vi "comm set rts.vi"(8 "error in (no error)":errorcluster, 11 "Comm Handle":u32) -> (0 "error out":errorcluster, 3 "dup Comm Handle":u32)   [LabVIEW 2017, in "lvserial.lvlib"]
doc: "Sends the RTS (RequestToSend) signal."
uses:
  lvserial.lvlib
  lvserial.dll
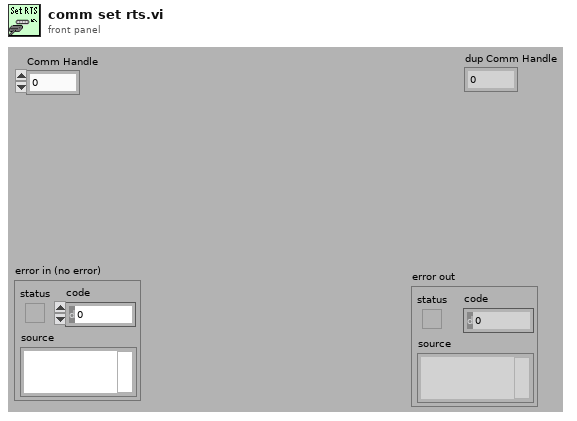
[diagram p1: front panel]
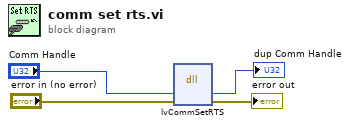
[diagram p0: block diagram]
diagram:
  n1 = dll-call lib="lvserial.dll" fn="lvCommSetRTS"("hComm"="Comm Handle", "error in (no error)"="error in (no error)") -> ("hComm"=→"dup Comm Handle":u32, "error in (no error)"=→"error out":errorcluster)  [unwired: 3 in, 3 out]
